vi "Close Panel.vi"(8 "error in (no error)":errorcluster, 11 "Post Analysis in":refnum<class "Post Analysis.lvclass">) -> (0 "error out":errorcluster, 3 "Post Analysis out":refnum<class "Post Analysis.lvclass">)   [LabVIEW 2023, in "Data Analysis.lvlib" / "Post Analysis.lvlib" / "Post Analysis.lvclass"]
uses:
  Post Analysis.lvclass
  Post Analysis.lvclass/Post Analysis.ctl
  Subpanel-Abstract Messages/Close SP Msg/Close SP Msg.lvclass
  <vilib>/ActorFramework/Actor/Actor.lvclass
  <vilib>/ActorFramework/Stop Msg/Stop Msg.lvclass
  8442e179-9ec6-4cbf-92f5-62a3267c4a6a.vi
  C:/Program Files/National Instruments/LabVIEW 2023/vi.lib/ActorFramework/Actor/Actor.lvclass
  D:/eDCU LTT/VT LTT Project/Source Code/Data Analysis/Post Analysis/Post Analysis.lvclass
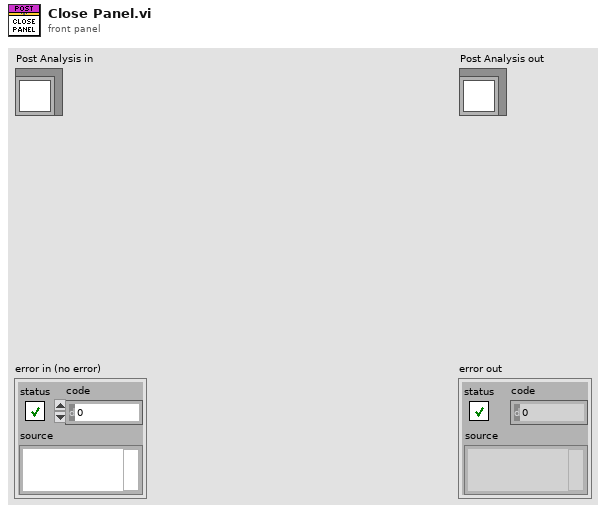
[diagram p1: front panel]
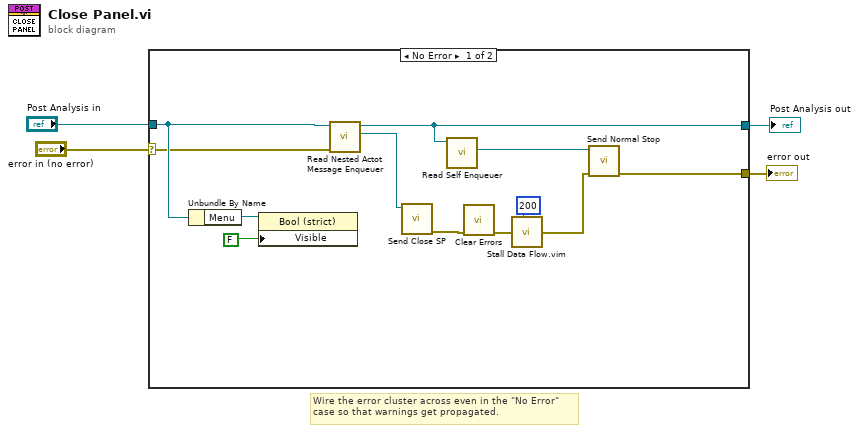
[diagram p0: block diagram]
diagram:
  # "Wire the error cluster across even in the \"No Error\"\ncase so that warnings get propagated."
  n1 = case shown="No Error" "error in (no error)" {
    selector: "error in (no error)" -> [w13 w18]
    tunnel: [w5 w18] -> w3
    tunnel: [w11 w17] -> w1
    tunnel: "Post Analysis in" -> [w14 w17]
    frame No Error {
      n2 = Unbundle By Name(w14) -> ("Menu"=w16:refnum<vi>)
      n3 = property class="Bool (strict)"(reference=w16, "Visible"=FALSE) -> ()  [unwired: 1 in, 2 out]
      n4 = call "Read Nested Actot Message Enqueuer.vi"("error in (no error)"=w13, "Post Analysis in"=w14) -> ("Actor Framework:Message Enqueuer"=w12:refnum<class "Message Enqueuer.lvclass">, "Post Analysis out"=w11:refnum<class "Post Analysis.lvclass">)  [unwired: 7 in, 1 out]
      n5 = call "Send Close SP.vi"("Message Enqueuer"=w12) -> ("error out"=w9:errorcluster)  [unwired: 9 in, 1 out]
      n6 = call <vilib>:"Read Self Enqueuer.vi"("Actor"=w11) -> ("Self Enqueuer"=w10:refnum<class "Message Enqueuer.lvclass">)  [unwired: 10 in]
      n7 = call <vilib>:"Clear Errors.vi"("error in (no error)"=w9) -> ("error out"=w8:errorcluster)  [unwired: 5 in, 1 out]
      n8 = call "Stall Data Flow.vim"("value in"=w8, "milliseconds to wait"=u32 200) -> ("value out"=w7:errorcluster)  [unwired: 1 out]
      n9 = call <vilib>:"Send Normal Stop.vi"("error in (no error)"=w7, "Message Enqueuer"=w10) -> ("error out"=w5:errorcluster)  [unwired: 9 in]
    }
    frame Error {
    }
  }
  "error out" <- w3
  "Post Analysis out" <- w1
